vi "FPGA-7842R-Reference.vi"(0 "Waveform Data":T3, 2 "Action":T4=enum."Exit", 7 "Manual Controls":T2={"Galvo 1 Position (I16)"=-280, "Galvo 2 Position (I16)"=-280, "X Axis Voltage (I16)"=0.0, "Y Axis Voltage (I16)"=0.0, "Z Axis Voltage (I16)"=0.0, "Res Mirror Amp (I16)"=0, "Res Mirror Mute"=FALSE, "Beam Blanking"=FALSE, "AOM (Pin 51 AO4)"=0}, 9 "Image Acquisition Parameters":T1={"Scan Type"=enum."Sample Scanning", "Scan Mode"=enum."XY", "Fast Axis Frequency (Hz)"=100.0, "Image Format"=128, "Line Accumulations"=1, "Number of Frames"=1.0, "Frames Per Capture"=1, "Frames Accumulations"=1, "Image Dimension (um)"=[], "Number of Z Steps"=1, "Z Steps Size (um)"=1.0, "Pixel Size (nm)"=[]} {"Image Format" items=["64 x 64"=64, "128 x 128"=128, "256 x 256"=256, "512 x 512"=512, "1024 x 1024"=1024, "2048 x 2048"=2048]}, 11 "Initialize":bool, 12 "Unused Axis Offset (I16)":i16) -> (15 "Initalized":bool)   [LabVIEW 2014]
uses:
  FPGA-7842R-Reference.ctl
  Waveform Data.ctl
  Manual Controls V2.ctl
  Type Defs/Image Acquisition Parameters.ctl
  <vilib>/FPGAPlugInAG/PCIe-7841R/niLvFpga_Open_PCIe-7841R.vi
  <vilib>/rvi/interface/common/dynamic/niFpgaDynamicAddResources.vi
  <vilib>/Utility/error.llb/Error Cluster From Error Code.vi
  <vilib>/rvi/errors/niLvFpgaAdjustHostInterfaceError.vi
  <vilib>/FPGAPlugInAG/Dynamic/niLvFpga_Run_Dynamic.vi
  <vilib>/FPGAPlugInAG/Dynamic/niLvFpga_Close_Dynamic.vi
  <vilib>/rvi/interface/nirviOpenFPGA/nirviOpenFPGA.xnode
  FPGA Bitfiles/MainSTEDFPGAProj_FPGATarget_WaveformandLaser_r4jCxZ5mzM0.lvbitx
  FPGA Target VIs/FPGA-7841R/Waveform and Laser Controls V3.vi
  <vilib>/rvi/interface/nirviReadWriteControl/nirviReadWriteControl.xnode
  <vilib>/rvi/interface/nirviMethod/nirviMethod.xnode
  <vilib>/rvi/interface/nirviCloseFPGA/nirviCloseFPGA.xnode
  NiFpgaLv.dll
  <vilib>/rvi/interface/Simulation/niFpgaSimulationCallBeginRW.vi
panel:
  # "XY"
  # "Z"
  # "Length"
  # "Height"
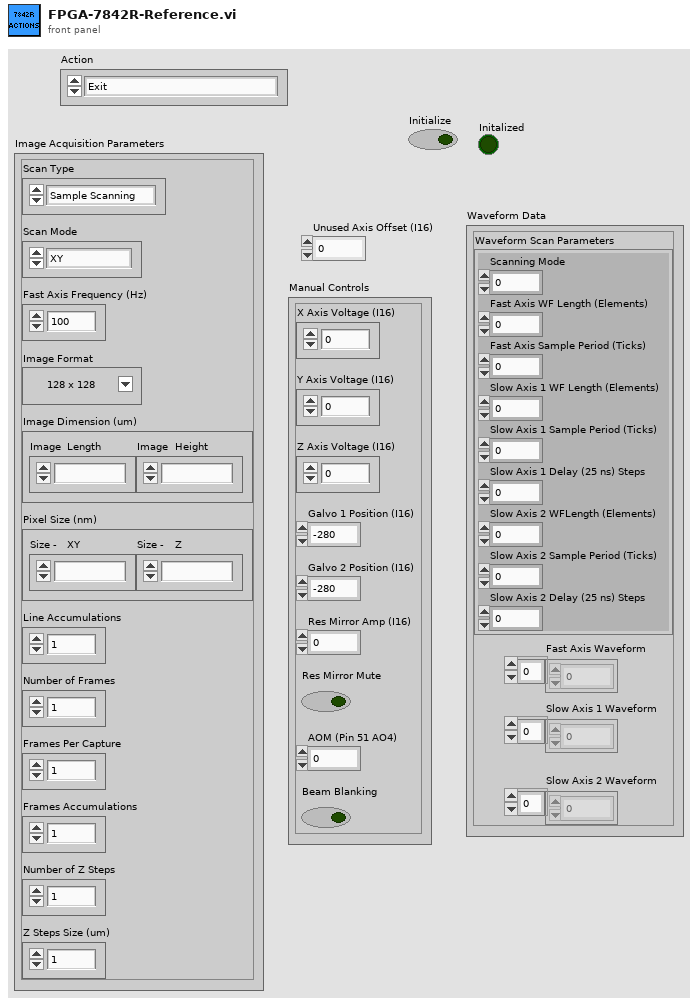
[diagram p1: front panel]
types:
  T1 = typedef "Image Acquisition Parameters.ctl" = cluster{"Scan Type":enum16{"Sample Scanning", "Beam Scanning"}, "Scan Mode":enum16{"XY", "XZ", "YZ", "XYZ"}, "Fast Axis Frequency (Hz)":dbl, "Image Format":u16, "Line Accumulations":u16, "Number of Frames":dbl, "Frames Per Capture":u16, "Frames Accumulations":u16, "Image Dimension (um)":dbl[], "Number of Z Steps":u8, "Z Steps Size (um)":dbl, "Pixel Size (nm)":dbl[]}
  T2 = typedef "Manual Controls V2.ctl" = cluster{"Galvo 1 Position (I16)":i16, "Galvo 2 Position (I16)":i16, "X Axis Voltage (I16)":dbl, "Y Axis Voltage (I16)":dbl, "Z Axis Voltage (I16)":dbl, "Res Mirror Amp (I16)":i16, "Res Mirror Mute":bool, "Beam Blanking":bool, "AOM (Pin 51 AO4)":i16}
  T3 = typedef "Waveform Data.ctl" = cluster{"Waveform Scan Parameters":cluster{"Scanning Mode":u8, "Fast Axis WF Length (Elements)":i32, "Fast Axis Sample Period (Ticks)":u32, "Slow Axis 1 WF Length (Elements)":i32, "Slow Axis 1 Sample Period (Ticks)":u32, "Slow Axis 1 Delay (25 ns) Steps":i32, "Slow Axis 2 WFLength (Elements)":i32, "Slow Axis 2 Sample Period (Ticks)":u32, "Slow Axis 2 Delay (25 ns) Steps":i32}, "Fast Axis Waveform":dbl[], "Slow Axis 1 Waveform":dbl[], "Slow Axis 2 Waveform":dbl[]}
  T4 = typedef "FPGA-7842R-Reference.ctl" = enum16{"Set STED AOM", "Unused Axis I16", "Exit", "Set Res Mirror", "Set Galvo", "Default", "Close FPGA", "Stop Waveforms", "Start Waveforms", "Initialize"}
  T5 = cluster{"Scanning Mode":u8, "Fast Axis WF Length (Elements)":i32, "Fast Axis Sample Period (Ticks)":u32, "Slow Axis 1 WF Length (Elements)":i32, "Slow Axis 1 Sample Period (Ticks)":u32, "Slow Axis 1 Delay (25 ns) Steps":i32, "Slow Axis 2 WFLength (Elements)":i32, "Slow Axis 2 Sample Period (Ticks)":u32, "Slow Axis 2 Delay (25 ns) Steps":i32}
  T6 = cluster{"Res Mirror Amp (I16)":i16, "Res Mirror Mute":bool}
  T7 = cluster{"AOM (Pin 51 AO4)":i16, "Beam Blanking":bool}
  T8 = typedef "Scan Parameters.ctl" = cluster{"Fast Axis Amplitude (V)":dbl, "Fast Axis Offset (V)":dbl, "Slow Axis Amplitude (V)":dbl, "Slow Axis Offset (V) ":dbl, "Slow Axis Max Velocity (V/s)":dbl, "Slow Axis 1 Delay (25 ns) Steps":i32, "Slow Axis 2 Delay (25 ns) Steps":i32, "Stage X Axis Offset (V)":dbl, "Stage Y Axis Offset (V)":dbl, "Stage Z Axis Offset (V)":dbl, "Galvo 1 Offset (V)":dbl, "Galvo 2 Offset (V)":dbl, "Last Scan Mode":enum16{"XY", "XZ", "YZ", "XYZ"}, "Current Scan Mode":enum16{"XY", "XZ", "YZ", "XYZ"}, "Fly Back Lines":u16, "Linear Ramp End":u32, "Z Step Size (I16)":i16, "Z Start Position (I16)":i16}
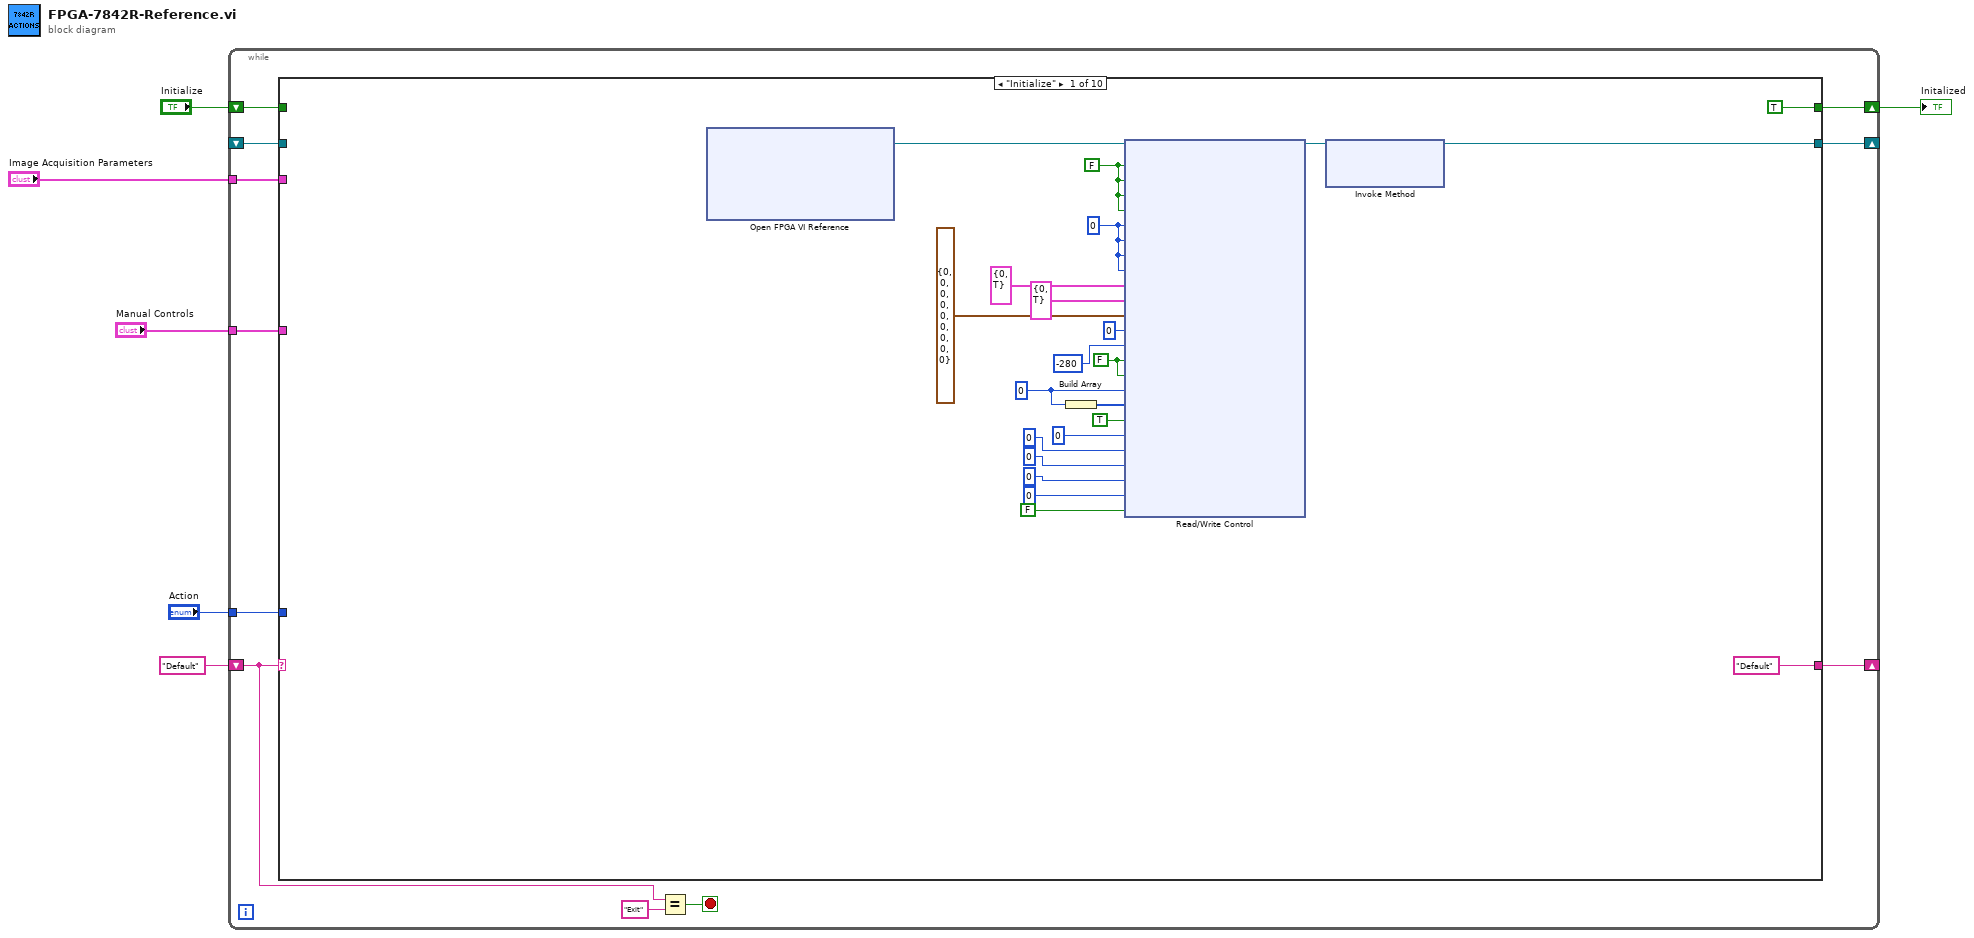
[diagram p0: block diagram]
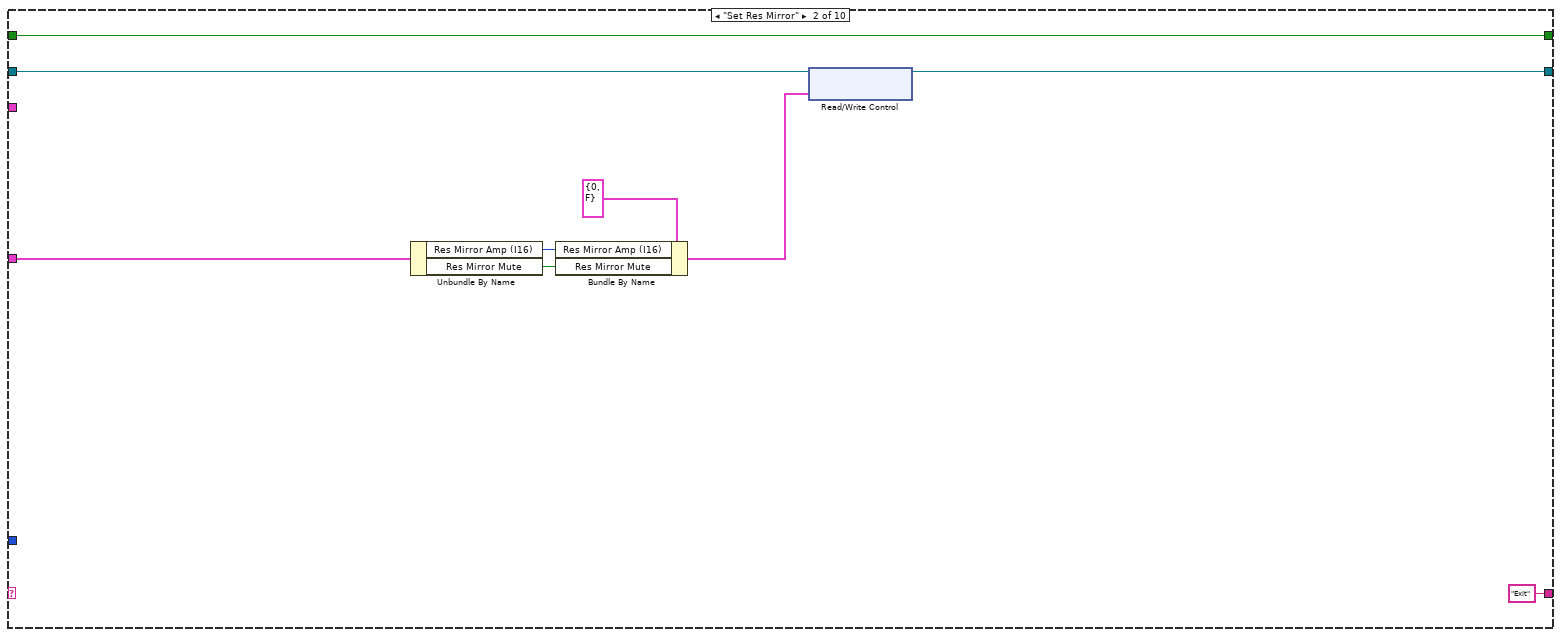
[diagram p2: hidden frame]
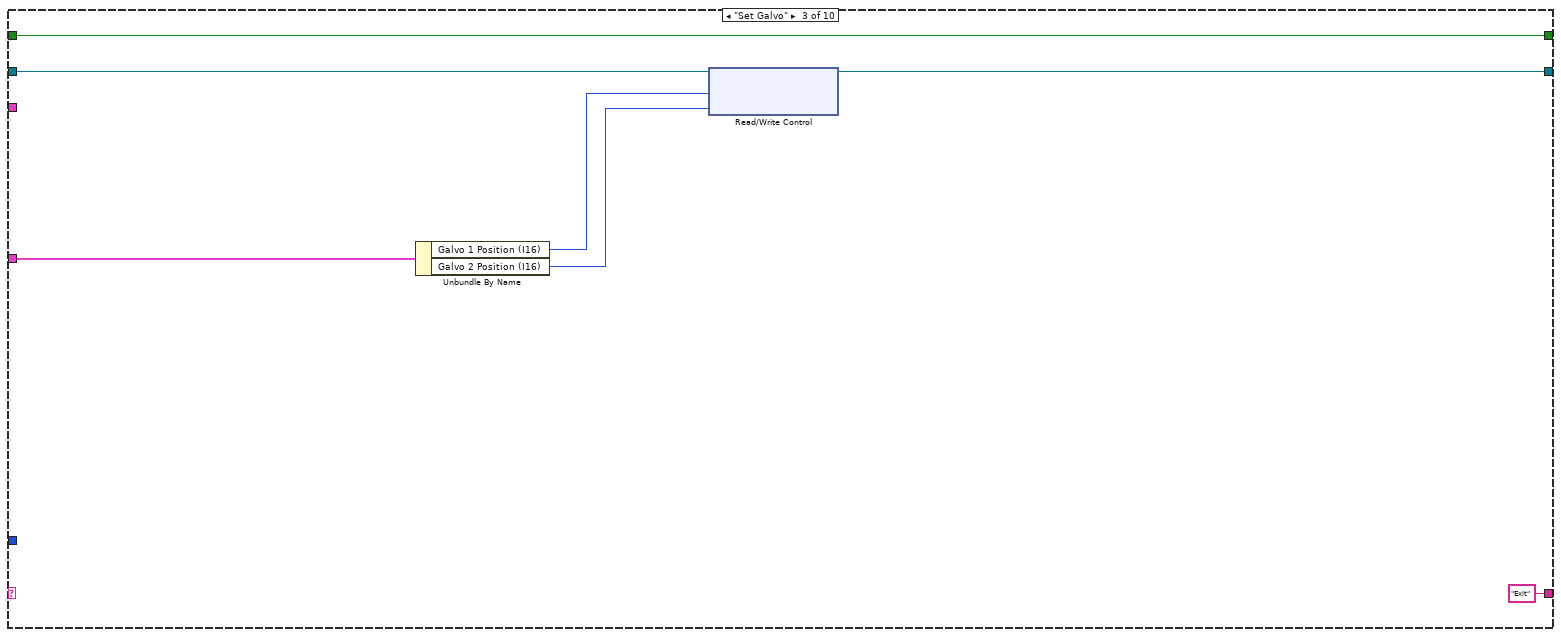
[diagram p3: hidden frame]
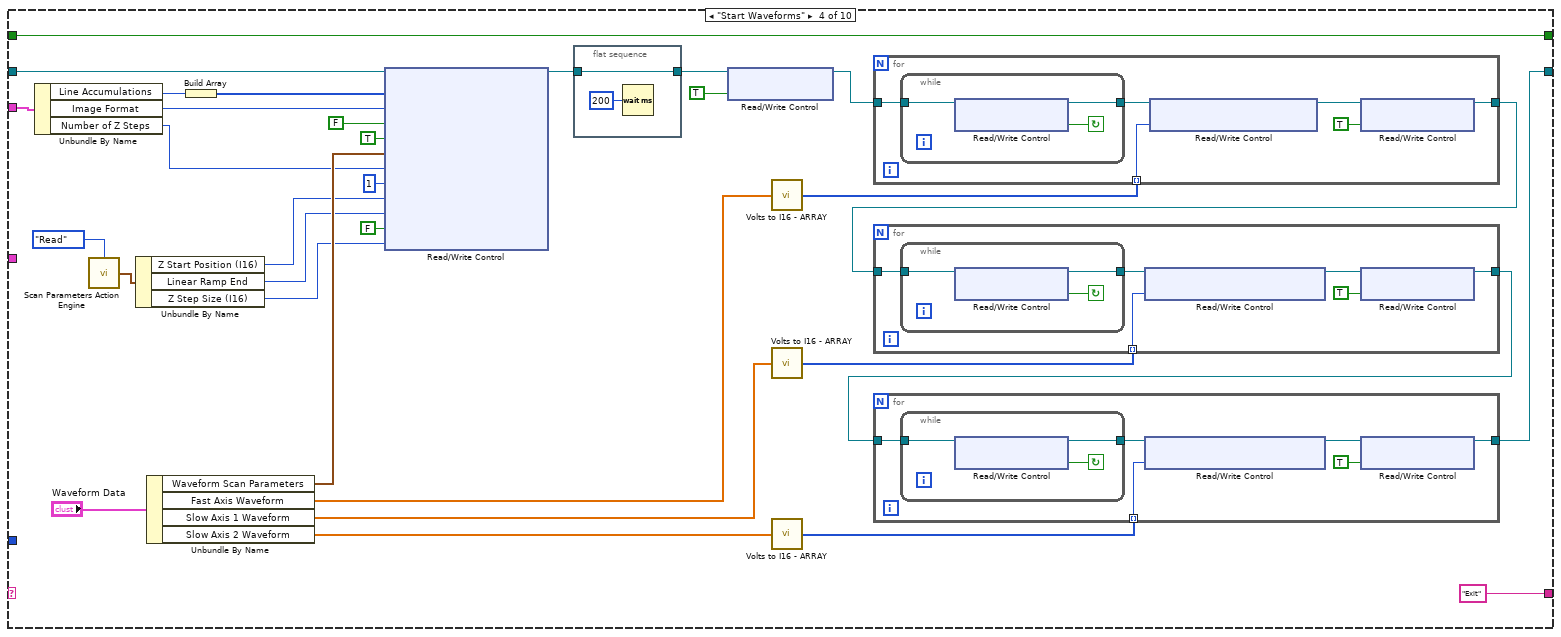
[diagram p4: hidden frame]
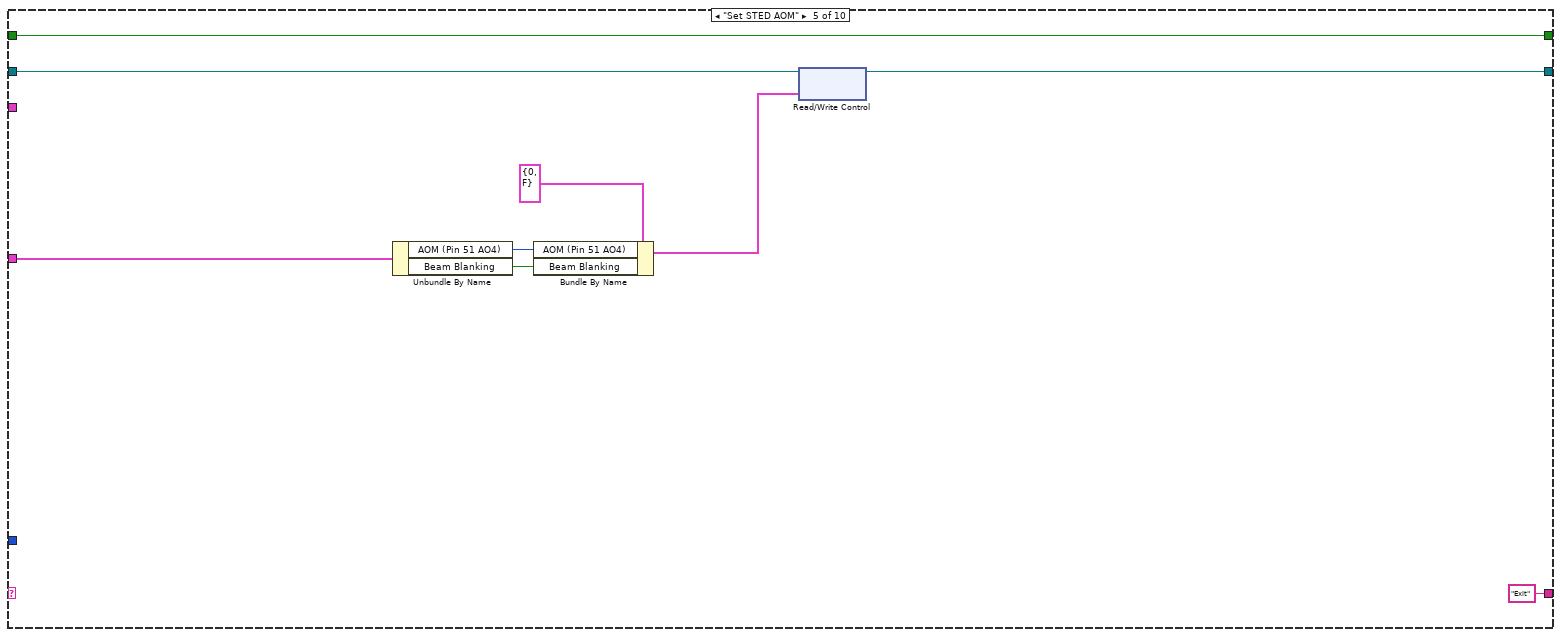
[diagram p5: hidden frame]
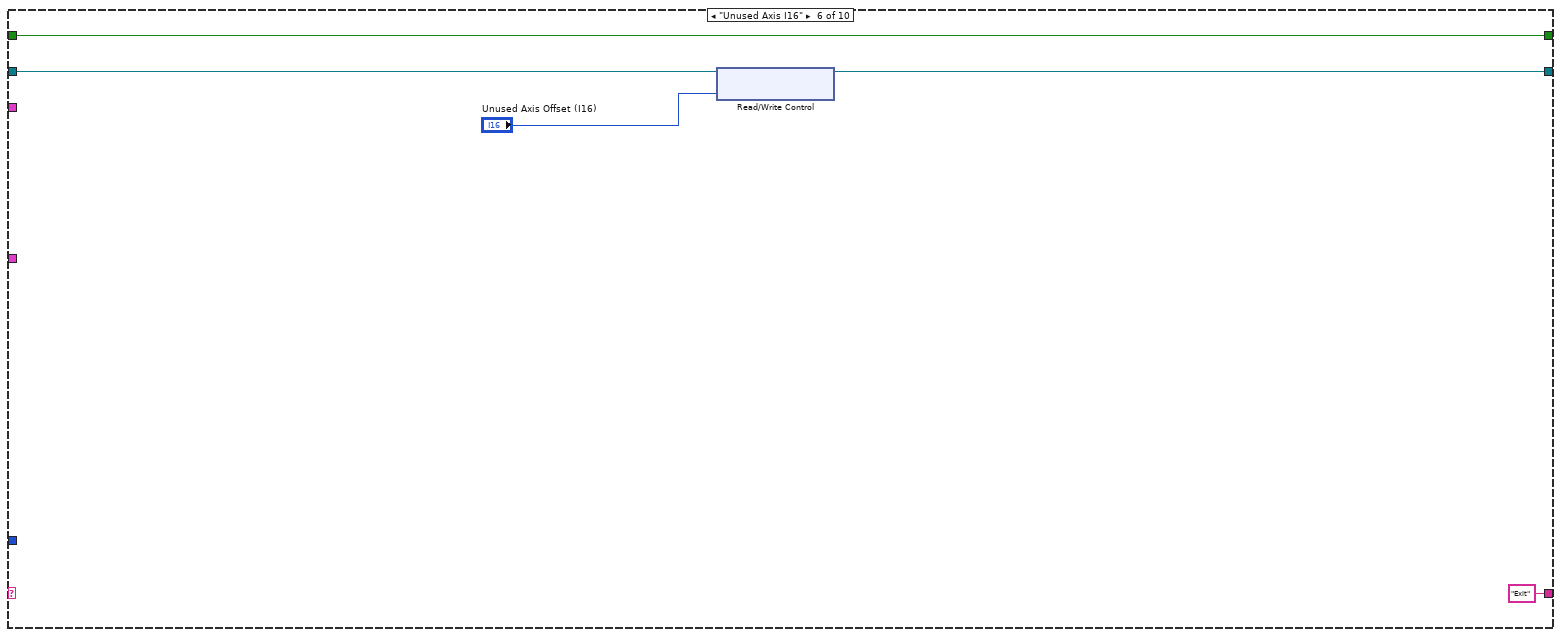
[diagram p6: hidden frame]
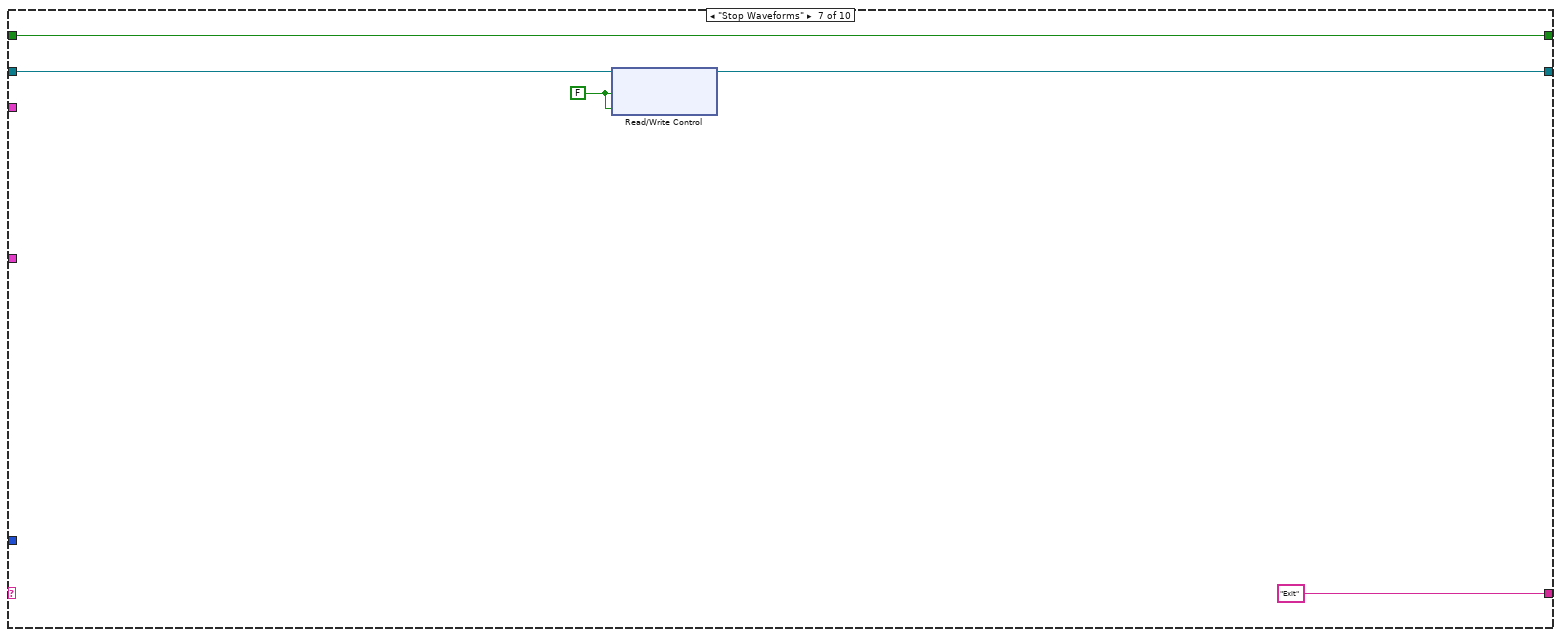
[diagram p7: hidden frame]
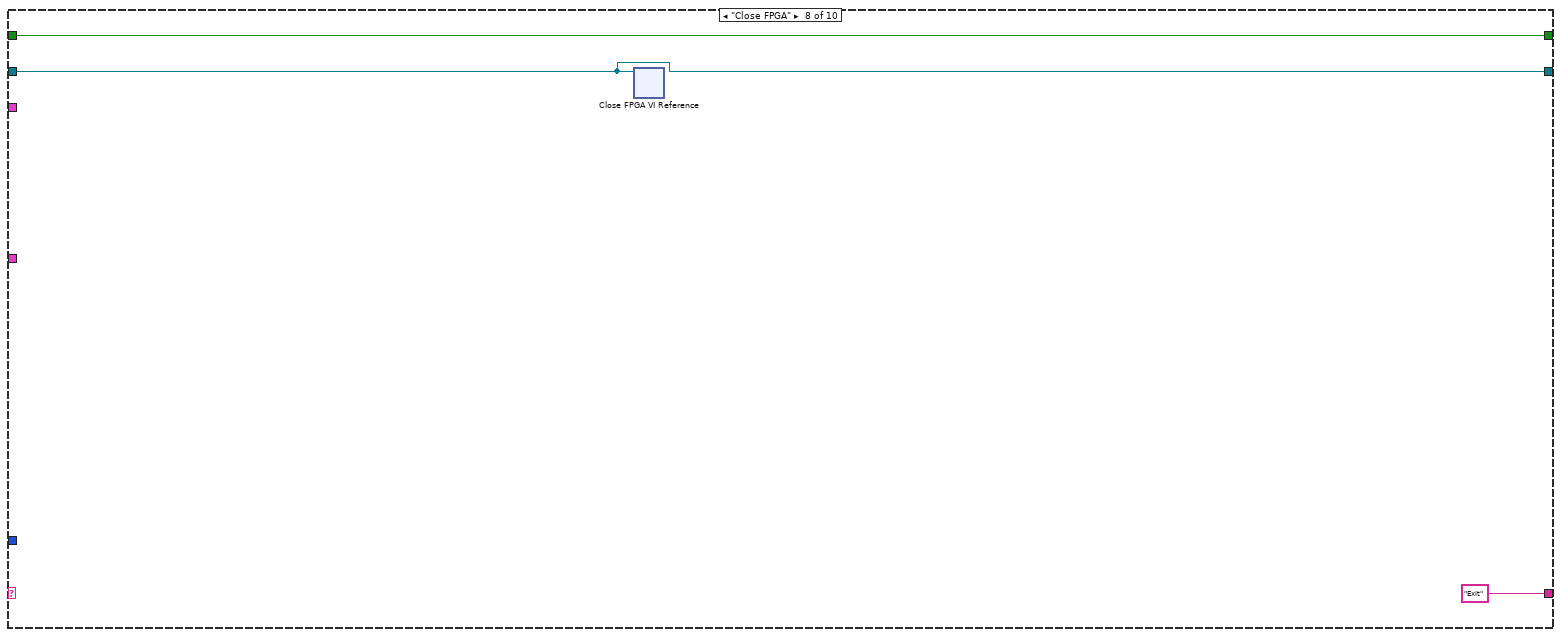
[diagram p8: hidden frame]
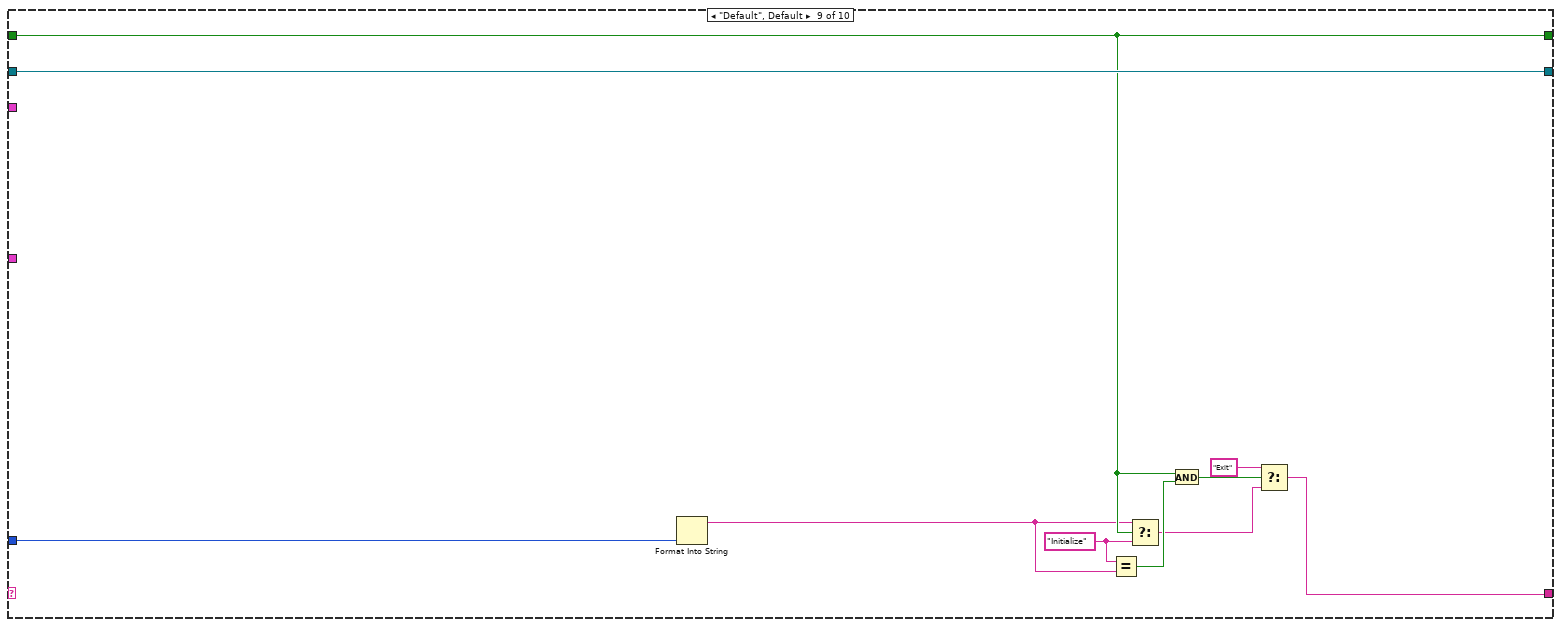
[diagram p9: hidden frame]
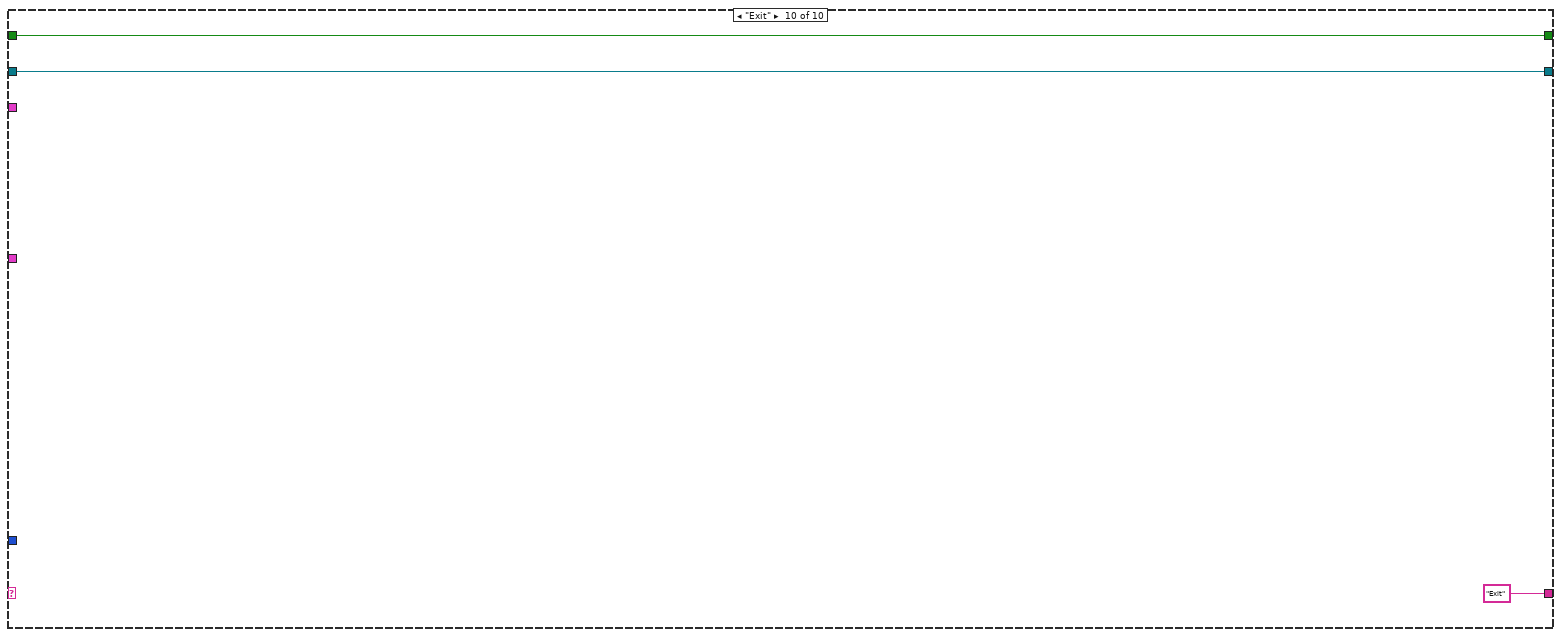
[diagram p10: hidden frame]
diagram:
  n1 = while {
    shift-right: [w17] -> _
    shift-left: _ -> [w16]
    shift-right: [w14] -> _
    shift-left: "Default" -> [w13]
    tunnel: "Action" -> [w15]
    shift-right: [w10] -> w3
    shift-left: "Initialize" -> [w9]
    tunnel: "Manual Controls" -> [w8]
    tunnel: "Image Acquisition Parameters" -> [w7]
    stop <- w11 stop-if-true
    n2 = case shown="\"Initialize\"" w13 {
      tunnel: [w29 w45 w52 w75 w124 w127 w134 w136 w148 w150] -> w17
      tunnel: w16 -> [_ w46 w53 w78 w125 w128 w135 w136 w148 w150]
      tunnel: w15 -> [_ _ _ _ _ _ _ _ w147 _]
      tunnel: ["Default" ("f") "Exit" ("f") "Exit" ("f") "Exit" ("f") "Exit" ("f") "Exit" ("f") "Exit" ("f") "Exit" ("f") w141 "Exit" ("f")] -> w14
      tunnel: [TRUE w48 w55 w80 w123 w130 w133 w138 w146 w151] -> w10
      tunnel: w9 -> [_ w48 w55 w80 w123 w130 w133 w138 w146 w151]
      tunnel: w8 -> [_ w44 w51 _ w119 _ _ _ _ _]
      tunnel: w7 -> [_ _ _ w68 _ _ _ _ _ _]
      frame "Initialize" {
        w25 = u16 0 ("Number of Lines")
        w27 = FALSE ("Reset Position Error")
        w39 = i16 0 ("Fast Axis Waveform Element")
        w38 = FALSE ("WF 1 Data Loaded")
        n3 = xnode "Open FPGA VI Reference"() -> ("FPGA VI Reference Out"=w28:refnum<k20>)  [unwired: 2 in, 1 out]
        n4 = Build Array(w25) -> (w24:u16[])
        n5 = xnode "Read/Write Control"("FPGA VI Reference In"=w28, "WF 1 Data Loaded"=w38, "WF 2 Data Loaded"=w38, "WF 3 Data Loaded"=w38, "Start Waveforms"=w38, "Fast Axis Waveform Element"=w39, "Slow Axis 1 Waveform Element"=w39, "Slow Axis 2 Waveform Element"=w39, "Unused Axis Offset"=w39, "775 AOM"=T7 {"AOM (Pin 51 AO4)"=0, "Beam Blanking"=TRUE}, "Resonant Mirror"=T6 {"Res Mirror Amp (I16)"=0, "Res Mirror Mute"=TRUE} ("Resoance Mirror"), "Waveform Scan Parameters"=T5 {"Scanning Mode"=0, "Fast Axis WF Length (Elements)"=0, "Fast Axis Sample Period (Ticks)"=0, "Slow Axis 1 WF Length (Elements)"=0, "Slow Axis 1 Sample Period (Ticks)"=0, "Slow Axis 1 Delay (25 ns) Steps"=0, "Slow Axis 2 WFLength (Elements)"=0, "Slow Axis 2 Sample Period (Ticks)"=0, "Slow Axis 2 Delay (25 ns) Steps"=0}, "Galvo 2 Position (I16)"=i16 0, "Galvo 1 Position (I16)"=i16 -280, "Reset Position Error"=w27, "Frame Trigger"=w27, "Number of Lines"=w25, "Accums Per Line"=w24, "Stop Sync Signal"=TRUE, "Z Step Size (I16)"=i16 0, "Number of Z Steps"=u8 0, "Frames Per Z Step"=u8 0, "Z Stack Start Position (I16)"=i16 0, "End of Linear Ramp"=u32 0, "End Linear Ramp"=FALSE) -> ("FPGA VI Reference Out"=w34:refnum<k20>)  [unwired: 1 in, 1 out]
        n6 = xnode "Invoke Method"("FPGA VI Reference In"=w34) -> ("FPGA VI Reference Out"=w29:refnum<k20>)  [unwired: 2 in, 1 out]
      }
      frame "Set Res Mirror" {
        n7 = Unbundle By Name(w44) -> ("Res Mirror Amp (I16)"=w43:i16, "Res Mirror Mute"=w42:bool)
        n8 = Bundle By Name(cluster=T6 {"Res Mirror Amp (I16)"=0, "Res Mirror Mute"=FALSE} ("Resoance Mirror"), "Res Mirror Amp (I16)"=w43, "Res Mirror Mute"=w42) -> (w40:T6)
        n9 = xnode "Read/Write Control"("FPGA VI Reference In"=w46, "Resonant Mirror"=w40) -> ("FPGA VI Reference Out"=w45:refnum<k20>)  [unwired: 1 in, 1 out]
      }
      frame "Set Galvo" {
        n10 = Unbundle By Name(w51) -> ("Galvo 1 Position (I16)"=w50:i16, "Galvo 2 Position (I16)"=w49:i16)
        n11 = xnode "Read/Write Control"("FPGA VI Reference In"=w53, "Galvo 1 Position (I16)"=w50, "Galvo 2 Position (I16)"=w49) -> ("FPGA VI Reference Out"=w52:refnum<k20>)  [unwired: 1 in, 1 out]
      }
      frame "Start Waveforms" {
        n12 = Unbundle By Name(w68) -> ("Line Accumulations"=w66:u16, "Image Format"=w67:u16, "Number of Z Steps"=w57:u8)
        n13 = call "Scan Parameters Action Engine.vi"("Action"=enum16{"Read", "Write"}."Read") -> ("Scan Parameters OUT"=w61:T8)  [unwired: 14 in]
        n14 = Unbundle By Name(w61) -> ("Z Start Position (I16)"=w59:i16, "Linear Ramp End"=w60:u32, "Z Step Size (I16)"=w56:i16)
        n15 = Unbundle By Name("Waveform Data") -> ("Waveform Scan Parameters"=w69:T5, "Fast Axis Waveform"=w82:dbl[], "Slow Axis 1 Waveform"=w74:dbl[], "Slow Axis 2 Waveform"=w81:dbl[])
        n16 = Build Array(w66) -> (w65:u16[])
        n17 = xnode "Read/Write Control"("FPGA VI Reference In"=w78, "Accums Per Line"=w65, "Number of Lines"=w67, "Frame Trigger"=FALSE, "Stop Sync Signal"=TRUE, "Waveform Scan Parameters"=w69, "Number of Z Steps"=w57, "Frames Per Z Step"=u8 1, "Z Stack Start Position (I16)"=w59, "End of Linear Ramp"=w60, "End Linear Ramp"=FALSE, "Z Step Size (I16)"=w56) -> ("FPGA VI Reference Out"=w76:refnum<k20>)  [unwired: 1 in, 1 out]
        n18 = flat-sequence {
          tunnel: [w89] -> w77
          tunnel: w76 -> [w89]
          frame #0 {
            n19 = Wait (ms)(milliseconds to wait=u32 200) -> ()  [unwired: 1 out]
          }
        }
        n20 = xnode "Read/Write Control"("FPGA VI Reference In"=w77, "Start Waveforms"=TRUE) -> ("FPGA VI Reference Out"=w83:refnum<k20>)  [unwired: 1 in, 1 out]
        n21 = call "Volts to I16 - ARRAY.vi"("Voltage (V)"=w82) -> ("I16"=w87:i16[])  [unwired: 14 in]
        n22 = call "Volts to I16 - ARRAY.vi"("Voltage (V)"=w74) -> ("I16"=w72:i16[])  [unwired: 14 in]
        n23 = call "Volts to I16 - ARRAY.vi"("Voltage (V)"=w81) -> ("I16"=w73:i16[])  [unwired: 14 in]
        n24 = for {
          tunnel: w83 -> [w112]
          tunnel: [w110] -> w86
          tunnel: w87 -> [w108] mode=indexing
          n25 = while {
            tunnel: w112 -> [w116]
            tunnel: [w115] -> w111
            stop <- w114 continue-if-true
            n26 = xnode "Read/Write Control"("FPGA VI Reference In"=w116) -> ("FPGA VI Reference Out"=w115:refnum<k20>, "WF 1 Data Loaded"=w114:bool)  [unwired: 1 in, 1 out]
          }
          n27 = xnode "Read/Write Control"("FPGA VI Reference In"=w111, "Fast Axis Waveform Element"=w108) -> ("FPGA VI Reference Out"=w113:refnum<k20>)  [unwired: 1 in, 1 out]
          n28 = xnode "Read/Write Control"("FPGA VI Reference In"=w113, "WF 1 Data Loaded"=TRUE ("Host Data Loaded")) -> ("FPGA VI Reference Out"=w110:refnum<k20>)  [unwired: 1 in, 1 out]
        }
        n29 = for {
          tunnel: w86 -> [w103]
          tunnel: [w101] -> w85
          tunnel: w72 -> [w99] mode=indexing
          n30 = while {
            tunnel: w103 -> [w107]
            tunnel: [w106] -> w102
            stop <- w105 continue-if-true
            n31 = xnode "Read/Write Control"("FPGA VI Reference In"=w107) -> ("FPGA VI Reference Out"=w106:refnum<k20>, "WF 2 Data Loaded"=w105:bool)  [unwired: 1 in, 1 out]
          }
          n32 = xnode "Read/Write Control"("FPGA VI Reference In"=w102, "Slow Axis 1 Waveform Element"=w99) -> ("FPGA VI Reference Out"=w104:refnum<k20>)  [unwired: 1 in, 1 out]
          n33 = xnode "Read/Write Control"("FPGA VI Reference In"=w104, "WF 2 Data Loaded"=TRUE ("Host Data Loaded")) -> ("FPGA VI Reference Out"=w101:refnum<k20>)  [unwired: 1 in, 1 out]
        }
        n34 = for {
          tunnel: w85 -> [w94]
          tunnel: [w92] -> w75
          tunnel: w73 -> [w90] mode=indexing
          n35 = while {
            tunnel: w94 -> [w98]
            tunnel: [w97] -> w93
            stop <- w96 continue-if-true
            n36 = xnode "Read/Write Control"("FPGA VI Reference In"=w98) -> ("FPGA VI Reference Out"=w97:refnum<k20>, "WF 3 Data Loaded"=w96:bool)  [unwired: 1 in, 1 out]
          }
          n37 = xnode "Read/Write Control"("FPGA VI Reference In"=w93, "Slow Axis 2 Waveform Element"=w90) -> ("FPGA VI Reference Out"=w95:refnum<k20>)  [unwired: 1 in, 1 out]
          n38 = xnode "Read/Write Control"("FPGA VI Reference In"=w95, "WF 3 Data Loaded"=TRUE ("Host Data Loaded")) -> ("FPGA VI Reference Out"=w92:refnum<k20>)  [unwired: 1 in, 1 out]
        }
      }
      frame "Set STED AOM" {
        n39 = Unbundle By Name(w119) -> ("AOM (Pin 51 AO4)"=w118:i16, "Beam Blanking"=w117:bool)
        n40 = Bundle By Name(cluster=T7 {"AOM (Pin 51 AO4)"=0, "Beam Blanking"=FALSE} ("775 AOM"), "AOM (Pin 51 AO4)"=w118, "Beam Blanking"=w117) -> (w120:T7)
        n41 = xnode "Read/Write Control"("FPGA VI Reference In"=w125, "775 AOM"=w120) -> ("FPGA VI Reference Out"=w124:refnum<k20>)  [unwired: 1 in, 1 out]
      }
      frame "Unused Axis I16" {
        n42 = xnode "Read/Write Control"("FPGA VI Reference In"=w128, "Unused Axis Offset"="Unused Axis Offset (I16)") -> ("FPGA VI Reference Out"=w127:refnum<k20>)  [unwired: 1 in, 1 out]
      }
      frame "Stop Waveforms" {
        w131 = FALSE ("Start Waveforms")
        n43 = xnode "Read/Write Control"("FPGA VI Reference In"=w135, "Start Waveforms"=w131, "Stop Sync Signal"=w131) -> ("FPGA VI Reference Out"=w134:refnum<k20>)  [unwired: 1 in, 1 out]
      }
      frame "Close FPGA" {
        n44 = xnode "Close FPGA VI Reference"("FPGA VI Reference In"=w136) -> ()  [unwired: 1 in, 1 out]
      }
      frame "Default", Default {
        w140 = "Initialize" ("f")
        n45 = Format Into String(w147) -> (resulting string=w139:string)  [unwired: 3 in, 1 out]
        n46 = Equal?(x=w140, y=w139) -> (x = y?=w145:bool)
        n47 = Select(t=w139, s=w146, f=w140) -> (s? t:f=w142:string)
        n48 = And(x=w146, y=w145) -> (x .and. y?=w144:bool)
        n49 = Select(t="Exit" ("y"), s=w144, f=w142) -> (s? t:f=w141:string)
      }
      frame "Exit" {
      }
    }
    n50 = Equal?(x=w13, y="Exit") -> (x = y?=w11:bool)
  }
  "Initalized" <- w3
